vi "Get MessageQ Status.vi"(7 "return elements? (F)":bool, 8 "error in (no error)":errorcluster, 11 "Process in":refnum<class "Process.lvclass">) -> (0 "error out":errorcluster, 1 "elements":T1[](array[typedef]), 2 "# elements in MessageQ":i32, 3 "Process out":refnum<class "Process.lvclass">)   [LabVIEW 2019, in "TelemetryAsync Engine.lvlib" / "Process.lvclass"]
uses:
  Process.lvclass
  TypeDefs/Message.ctl
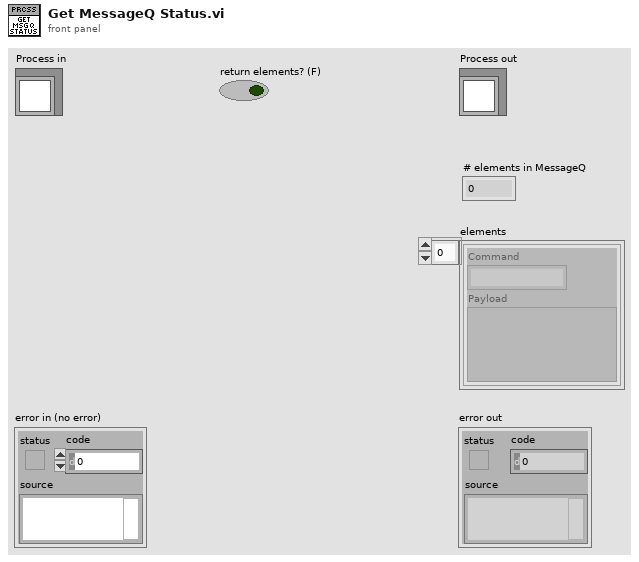
[diagram p1: front panel]
types:
  T1 = typedef "TelemetryAsync Engine.lvlib/Process.lvclass/Message.ctl" = cluster{"Command":string, "Payload":variant}
  T2 = typedef "TelemetryAsync Engine.lvlib/Process.lvclass/Process Lookup.ctl" = cluster{"Process ID":string, "MessageQ":refnum<queue>, "Update UE":refnum<user-event>}
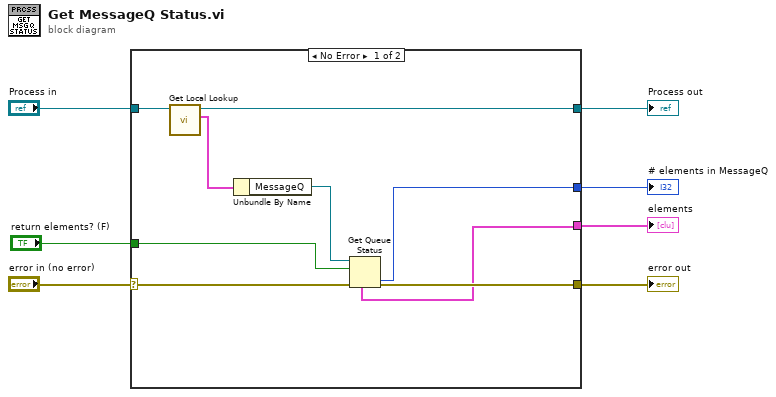
[diagram p0: block diagram]
diagram:
  n1 = case shown="No Error" "error in (no error)" {
    selector: "error in (no error)" -> [w14 w18]
    tunnel: [w11 w18] -> w6
    tunnel: [w8 w17] -> w4
    tunnel: "Process in" -> [w16 w17]
    tunnel: "return elements? (F)" -> [w12 _]
    tunnel: [w10 _] -> w2
    tunnel: [w9 _] -> w1
    frame No Error {
      n2 = call-dynamic "Get Local Lookup.vi"("Process in"=w16) -> ("Process Lookup"=w15:T2, "Process out"=w8:refnum<class "Process.lvclass">)  [unwired: 8 in, 1 out]
      n3 = Unbundle By Name(w15) -> ("MessageQ"=w13:refnum<queue>)
      n4 = Get Queue Status(queue=w13, return elements? (F)=w12, error in (no error)=w14) -> (error out=w11:errorcluster, # elements in queue=w10:i32, elements=w9:T1[])  [unwired: 5 out]
    }
    frame Error {
    }
  }
  "error out" <- w6
  "Process out" <- w4
  "# elements in MessageQ" <- w2
  "elements" <- w1
